vi "getParentClass.vi"(8 "error in (no error)":errorcluster, 11 "Class Ref":refnum<vi>) -> (0 "error out":errorcluster, 2 "Parent Class Name":string, 3 "Parent Class Ref":refnum<vi>)   [LabVIEW 2018, in "TestCase.lvclass"]
uses:
  TestCase.lvclass
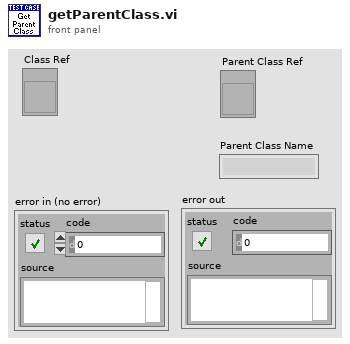
[diagram p1: front panel]
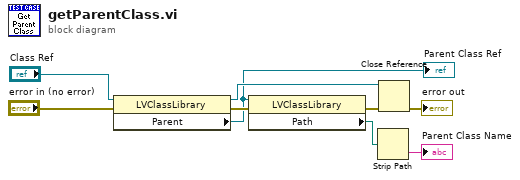
[diagram p0: block diagram]
diagram:
  n1 = property class="LVClassLibrary"(reference="Class Ref", error in="error in (no error)") -> (reference out=w7:refnum<vi>, error out=w9:errorcluster, "Parent"=w1:refnum<vi>)
  "Parent Class Ref" <- w1
  n2 = property class="LVClassLibrary"(reference=w1, error in=w9) -> (error out=w2:errorcluster, "Path"=w8:path)  [unwired: 1 out]
  n3 = Strip Path(path=w8) -> (name=→"Parent Class Name":string)  [unwired: 1 out]
  n4 = Close Reference(reference=w7, error in (no error)=w2) -> (error out=→"error out":errorcluster)
